vi "tsapp_show_channel_mapping_window.vi"(8 "error in (no error)":errorcluster caption="错误输入（无错误）", 11 "路径输入":path) -> (0 "error out":errorcluster caption="错误输出", 2 "function return":i32, 3 "路径输出":path)   [LabVIEW 2014]
doc: "TSAPI(s32)tsapp_show_hardware_configuration_window();"
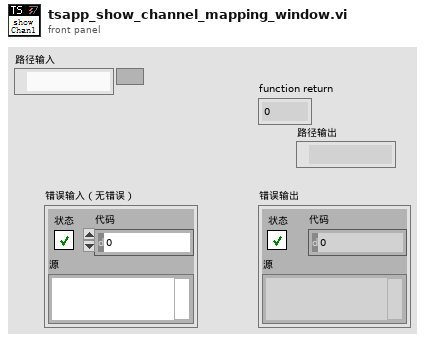
[diagram p1: front panel]
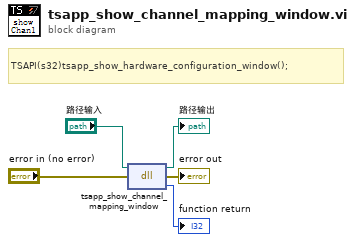
[diagram p0: block diagram]
diagram:
  # "TSAPI(s32)tsapp_show_hardware_configuration_window();"
  n1 = dll-call lib="D:/Program Files (x86)/TOSUN/TSMaster/bin/TSMaster.dll" fn="tsapp_show_channel_mapping_window"(path in="路径输入", error in="error in (no error)") -> (path out=→"路径输出":path, error out=→"error out":errorcluster, "返回类型"=→"function return":i32)  [unwired: 1 in]
